vi "FTPDownloadFile2.vi"() -> ()   [LabVIEW 2011, in "Medimatic.lvlib"]
uses:
  Medimatic.lvlib
  <vilib>/EvaluMation, LLC/FTP Toolkit/FTP Class/FTP.lvclass
panel:
  in  "FileName":string="FileVersion.txt"
  out "error out":errorcluster
  in  "error in (no error)":errorcluster
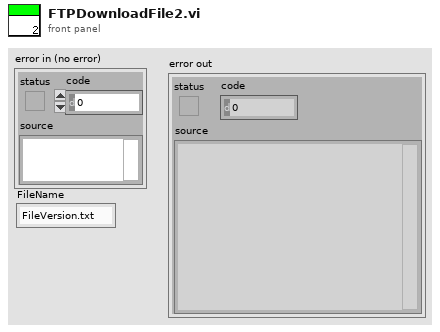
[diagram p1: front panel]
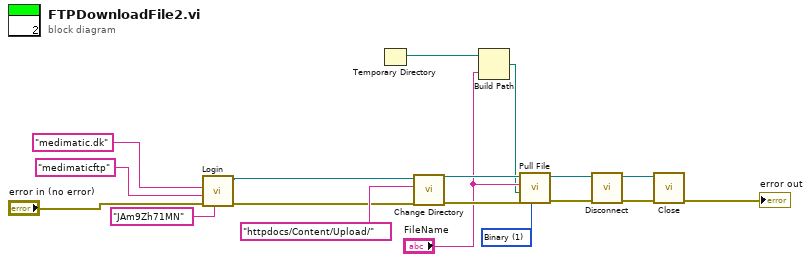
[diagram p0: block diagram]
diagram:
  w6 = u16 1 items=["ASCII", "Binary"] ("Type (Binary)")
  n1 = call <vilib>:"Login.vi"("passWord"="JAm9Zh71MN", "error in (no error)"="error in (no error)", "userName"="medimaticftp", "address"="medimatic.dk") -> ("error out"=w13:errorcluster, "FTP out"=w5:refnum<class "FTP.lvclass">)  [unwired: 6 in]
  n2 = Temporary Directory() -> (w9:path)
  n3 = call <vilib>:"Change Directory.vi"("error in (no error)"=w13, "RemoteDirectory"="httpdocs/Content/Upload/", "FTP in"=w5) -> ("error out"=w14:errorcluster, "FTP out"=w10:refnum<class "FTP.lvclass">)  [unwired: 7 in]
  n4 = Build Path(base path=w9, name or relative path="FileName") -> (appended path=w7:path)
  n5 = call <vilib>:"Pull File.vi"("Type (Binary)"=w6, "error in (no error)"=w14, "Local FilePath"=w7, "FileName"="FileName", "FTP in"=w10) -> ("error out"=w3:errorcluster, "FTP out"=w4:refnum<class "FTP.lvclass">)  [unwired: 5 in]
  n6 = call <vilib>:"Disconnect.vi"("error in (no error)"=w3, "FTP in"=w4) -> ("error out"=w2:errorcluster, "FTP out"=w1:refnum<class "FTP.lvclass">)  [unwired: 8 in]
  n7 = call <vilib>:"Close.vi"("error in (no error)"=w2, "FTP in"=w1) -> ("error out"=→"error out":errorcluster)  [unwired: 9 in]
